vi "test Work Directory.vi"(8 "error in":errorcluster) -> (0 "error out":errorcluster)   [LabVIEW 2020, in "serenial.io-ase.test.lvlib"]
uses:
  serenial.io-ase.test.lvlib
  serenial.io-ase/ase/Start Call (Exe Name).vi
  <vilib>/addons/_JKI Toolkits/Caraya/classes/Assert/Assert Equal Value_Variant.vi
  <vilib>/addons/_JKI Toolkits/Caraya/classes/Test/Test.lvclass
  serenial.io-ase/ase/ase.lvclass
  <vilib>/addons/_JKI Toolkits/Caraya/classes/Assert/Assert.lvclass
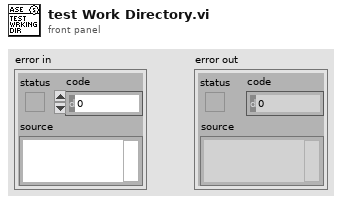
[diagram p1: front panel]
types:
  T1 = typedef "serenial.io-ase.lvlib/ase.lvclass/Event References.ctl" = cluster{"Standard Output":refnum<user-event>, "Standard Error":refnum<user-event>, "Did Exit":refnum<user-event>}
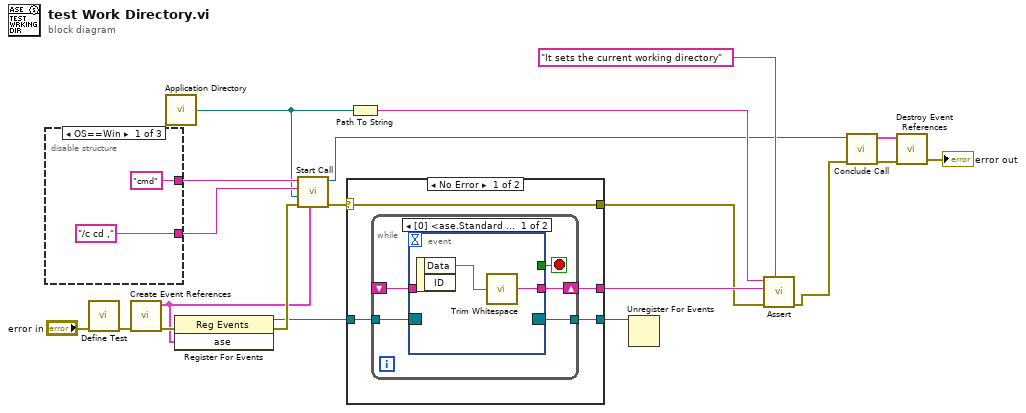
[diagram p0: block diagram]
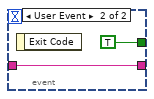
[diagram p2: hidden frame]
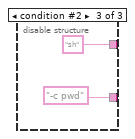
[diagram p5: hidden frame]
diagram:
  n1 = disable-structure "Conditional Disable Structure" shown="OS==Win" {
    disable-tunnel: ["cmd" _ "sh"] -> w9
    disable-tunnel: ["/c cd ," _ "-c pwd"] -> w14
    frame condition #0 (active) {
    }
    frame condition #1 {
    }
    frame condition #2 {
    }
  }
  n2 = call <vilib>:"Define Test.vi"("error in (no error)"="error in") -> ("error out"=w18:errorcluster)  [unwired: 10 in]
  n3 = call "Create Event References.vi"("error in"=w18) -> ("error out"=w19:errorcluster, "ase"=w6:T1)  [unwired: 9 in]
  n4 = call <vilib>:"Application Directory.vi"() -> ("Application Directory"=w8:path)
  n5 = register-events(error in=w19, w6) -> (reference out=w15:refnum<event-registration>, error out=w17:errorcluster)  [unwired: 1 in]
  n6 = call-poly "Start Call.vi"("Event References"=w6, "error in"=w17, "Working Directory (default <Not A Path> - System Default)"=w8, "Arguments"=w14, "Executable Name"=w9) -> ("error out"=w16:errorcluster, "New ASE Handle"=w5:refnum<class "ase.lvclass">)  [unwired: 5 in]
  n7 = case shown="No Error" w16 {
    selector: w16 -> [w28 w39]
    tunnel: w15 -> [w27 w38]
    tunnel: [w26 _] -> w11
    tunnel: [w25 w38] -> w13
    tunnel: [w28 w39] -> w7
    frame No Error {
      n8 = while {
        tunnel: w27 -> [w33]
        tunnel: [w31] -> w25
        shift-right: [w30] -> w26
        shift-left: _ -> [w29]
        stop <- w32 stop-if-true
        n9 = event shown="[0] <ase.Standard Output>: User Event" {
          selector: w33 -> [_ _]
          dyn-events: [_ _] -> w31
          timeout: _ -> [_ _]
          tunnel: [_ TRUE] -> w32
          tunnel: [w34 w36] -> w30
          tunnel: w29 -> [_ w36]
          event User Event {
            n10 = event-data() -> ("Data"=w35:string)  [unwired: 1 in, 1 out]
            n11 = call <vilib>:"Trim Whitespace.vi"("string"=w35) -> ("trimmed string"=w34:string)  [unwired: 1 in]
          }
          event User Event {
            n12 = event-data() -> ()  [unwired: 1 in, 1 out]
          }
        }
      }
    }
    frame Error {
    }
  }
  n13 = Path To String(path=w8) -> (string=w12:string)
  n14 = Unregister For Events(event registration refnum=w13) -> ()  [unwired: 1 in, 1 out]
  n15 = call-poly <vilib>:"Assert.vi"("Label"="It sets the current working directory", "error in (no error)"=w7, "Y"=w11, "X"=w12) -> ("error out"=w4:errorcluster)  [unwired: 7 in]
  n16 = call "Conclude Call.vi"("error in"=w4, "ASE Handle"=w5) -> ("error out"=w3:errorcluster, "Event References"=w1:T1)  [unwired: 7 in, 1 out]
  n17 = call "Destroy Event References.vi"("error in"=w3, "Event References"=w1) -> ("error out"=→"error out":errorcluster)  [unwired: 9 in]
